vi "test btn dialog with tmo.vi"() -> ()   [LabVIEW 2017]
panel:
  out "true":bool
  out "T button?":bool
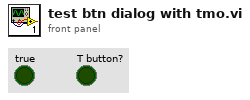
[diagram p1: front panel]
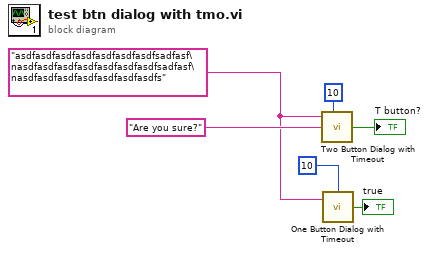
[diagram p0: block diagram]
diagram:
  w3 = "asdfasdfasdfasdfasdfasdfasdfsadfasf\nasdfasdfasdfasdfasdfasdfasdfsadfasf\nasdfasdfasdfasdfasdfasdfasdfs" ("Text")
  n1 = call "Two Button Dialog with Timeout.vi"("message"=w3, "T Timeout(-1 s)"=10, "T button name (\"OK\")"="Are you sure?" ("T button name (\"OK\")")) -> ("T button?"=→"T button?":bool)  [unwired: 2 in]
  n2 = call "One Button Dialog with Timeout.vi"("Btn Timeout(-1 s)"=10, "message"=w3) -> ("true"=→"true":bool)  [unwired: 1 in]
